vi "Get Aircraft GPS.vi"(8 "Error In":errorcluster, 11 "Aircraft ID":u8) -> (0 "Error Out":errorcluster, 3 "Aircraft GPS Data Out":T1)   [LabVIEW 2014]
uses:
  Controls/Aircraft GPS Data.ctl
  Controls/GPS Fix Type.ctl
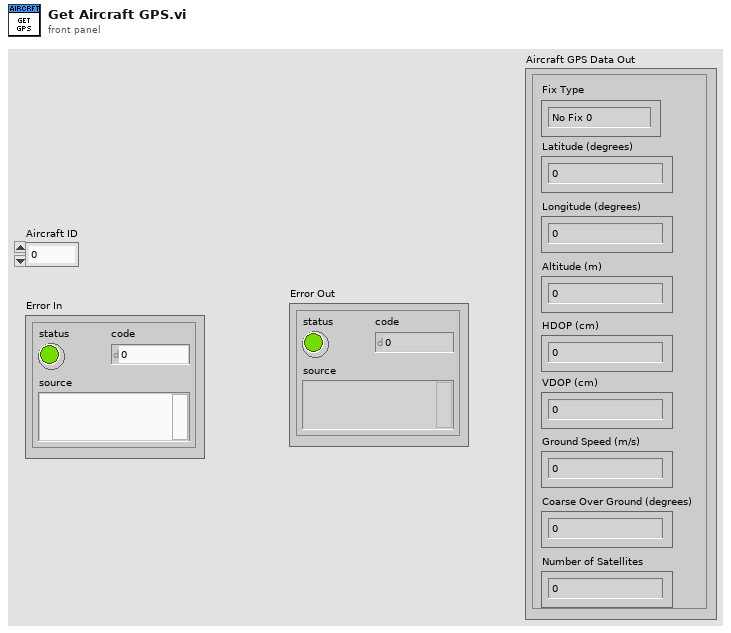
[diagram p1: front panel]
types:
  T1 = typedef "Aircraft GPS Data.ctl" = cluster{"Latitude (degrees)":dbl, "Longitude (degrees)":dbl, "Altitude (m)":dbl, "Fix Type":T2, "HDOP (cm)":u16, "VDOP (cm)":u16, "Ground Speed (m/s)":dbl, "Coarse Over Ground (degrees)":u16, "Number of Satellites":u8}
  T2 = typedef "GPS Fix Type.ctl" = enum16{"No Fix 0", "No Fix 1", "2D Fix", "3D Fix", "DGPS", "RTK"}
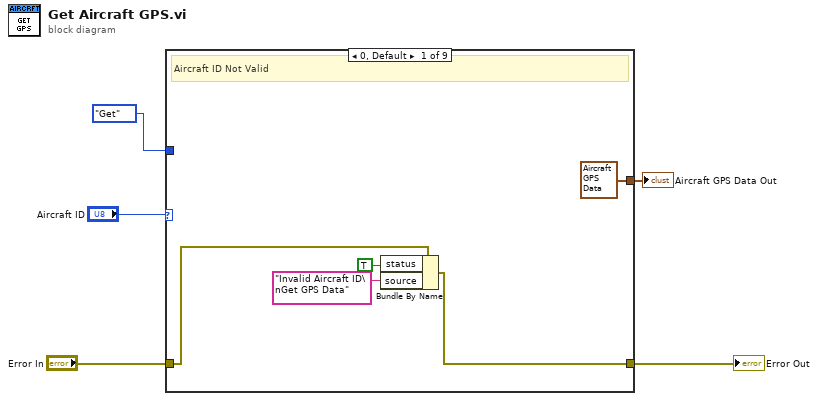
[diagram p0: block diagram]
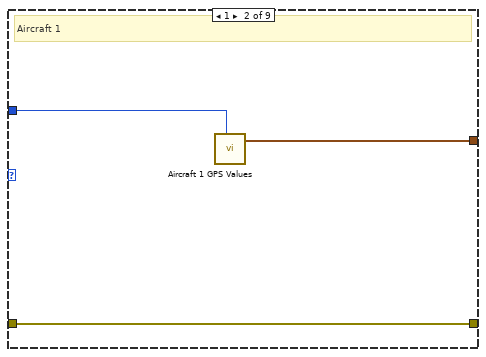
[diagram p2: hidden frame]
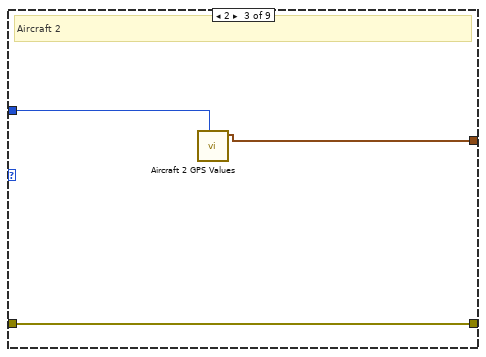
[diagram p3: hidden frame]
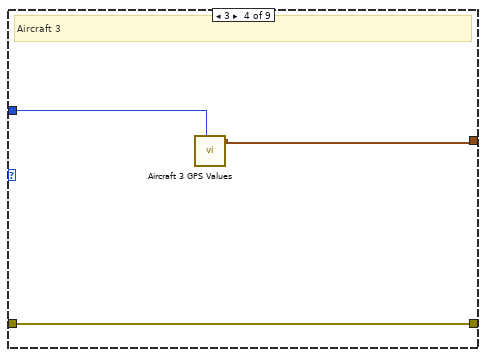
[diagram p4: hidden frame]
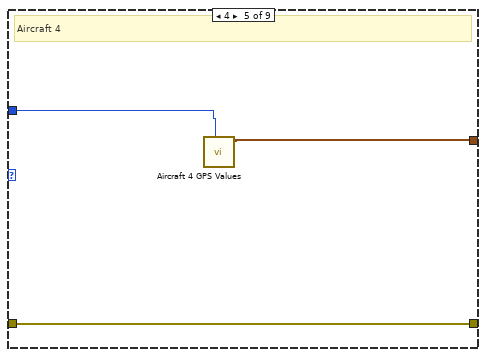
[diagram p5: hidden frame]
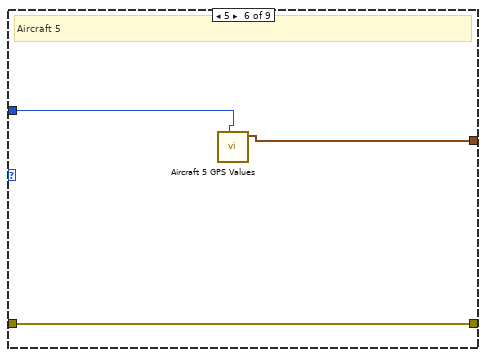
[diagram p6: hidden frame]
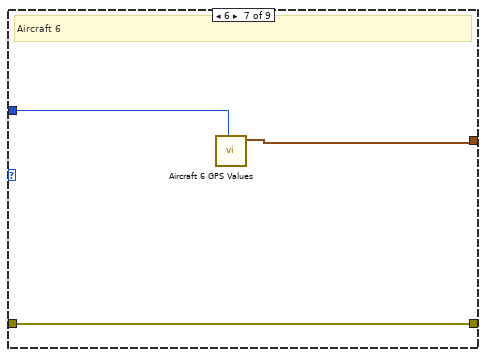
[diagram p7: hidden frame]
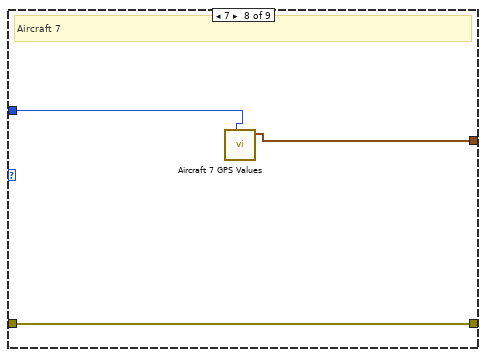
[diagram p8: hidden frame]
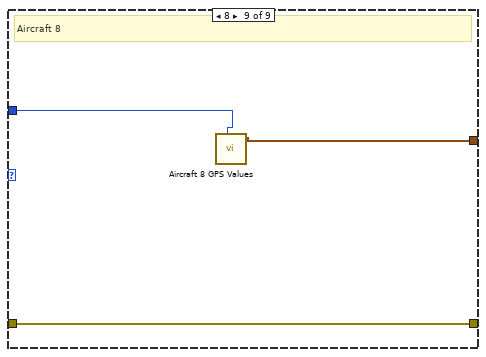
[diagram p9: hidden frame]
diagram:
  n1 = case shown="0, Default" "Aircraft ID" {
    tunnel: [T1 {"Latitude (degrees)"=0.0, "Longitude (degrees)"=0.0, "Altitude (m)"=0.0, "Fix Type"=enum."No Fix 0", "HDOP (cm)"=0, "VDOP (cm)"=0, "Ground Speed (m/s)"=0.0, "Coarse Over Ground (degrees)"=0, "Number of Satellites"=0} ("Aircraft GPS Data Out") w11 w15 w18 w21 w24 w27 w30 w33] -> w1
    tunnel: [w9 w13 w16 w19 w22 w25 w28 w31 w34] -> w4
    tunnel: "Error In" -> [w10 w13 w16 w19 w22 w25 w28 w31 w34]
    tunnel: enum16{"Get", "Set"}."Get" ("Method") -> [_ w12 w14 w17 w20 w23 w26 w29 w32]
    frame 0, Default {
      # "Aircraft ID Not Valid"
      n2 = Bundle By Name(cluster=w10, "status"=TRUE, "source"="Invalid Aircraft ID\nGet GPS Data") -> (w9:errorcluster)
    }
    frame 1 {
      # "Aircraft 1"
      n3 = call "Aircraft 1 GPS Values .vi"("Method"=w12) -> ("Aircraft GPS Data Out"=w11:T1)  [unwired: 10 in]
    }
    frame 2 {
      # "Aircraft 2"
      n4 = call "Aircraft 2 GPS Values .vi"("Method"=w14) -> ("Aircraft GPS Data Out"=w15:T1)  [unwired: 10 in]
    }
    frame 3 {
      # "Aircraft 3"
      n5 = call "Aircraft 3 GPS Values .vi"("Method"=w17) -> ("Aircraft GPS Data Out"=w18:T1)  [unwired: 10 in]
    }
    frame 4 {
      # "Aircraft 4"
      n6 = call "Aircraft 4 GPS Values .vi"("Method"=w20) -> ("Aircraft GPS Data Out"=w21:T1)  [unwired: 10 in]
    }
    frame 5 {
      # "Aircraft 5"
      n7 = call "Aircraft 5 GPS Values .vi"("Method"=w23) -> ("Aircraft GPS Data Out"=w24:T1)  [unwired: 10 in]
    }
    frame 6 {
      # "Aircraft 6"
      n8 = call "Aircraft 6 GPS Values .vi"("Method"=w26) -> ("Aircraft GPS Data Out"=w27:T1)  [unwired: 10 in]
    }
    frame 7 {
      # "Aircraft 7"
      n9 = call "Aircraft 7 GPS Values .vi"("Method"=w29) -> ("Aircraft GPS Data Out"=w30:T1)  [unwired: 10 in]
    }
    frame 8 {
      # "Aircraft 8"
      n10 = call "Aircraft 8 GPS Values .vi"("Method"=w32) -> ("Aircraft GPS Data Out"=w33:T1)  [unwired: 10 in]
    }
  }
  "Error Out" <- w4
  "Aircraft GPS Data Out" <- w1
